vi "1_9.vi"() -> ()   [LabVIEW 2020]
panel:
  in  "Lower limit":dbl(knob) scale=0.0..1000.0
  out "Number In Range?":bool
  in  "Upper limit":dbl(knob) scale=0.0..1000.0
  in  "Temp":dbl(slide) scale=0.0..1000.0
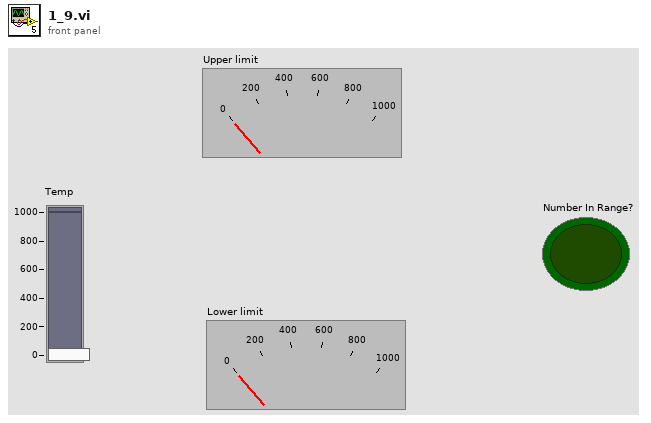
[diagram p1: front panel]
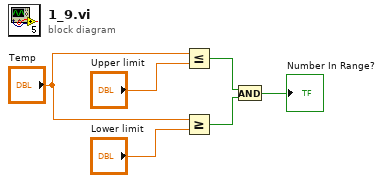
[diagram p0: block diagram]
diagram:
  n1 = Less Or Equal?(x="Temp", y="Upper limit") -> (x <= y?=w1:bool)
  n2 = Greater Or Equal?(x="Temp", y="Lower limit") -> (x >= y?=w6:bool)
  n3 = And(x=w1, y=w6) -> (x .and. y?=→"Number In Range?":bool)
